vi "Write Loop.vi"(7 "Enum - Menu":enum16{"INIT", "WRITE", "RE-INIT", "CLOSE"}(ring), 8 "error in (no error)":errorcluster, 11 "Uplink Packet":T1) -> (0 "error out":errorcluster)   [LabVIEW 2025]
panel:
  out "connection ID":refnum<k16>
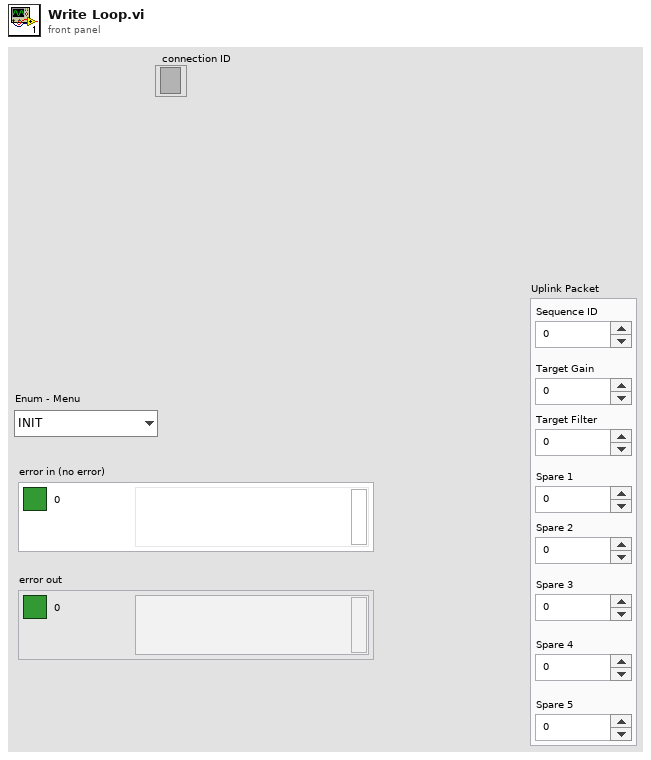
[diagram p1: front panel]
types:
  T1 = cluster{"Sequence ID":u32, "Target Gain":u32, "Target Filter":u32, "Spare 1":u32, "Spare 2":u32, "Spare 3":u32, "Spare 4":u32, "Spare 5":u32}
  T2 = enum16{"big-endian, network order", "native, host order", "little-endian"}
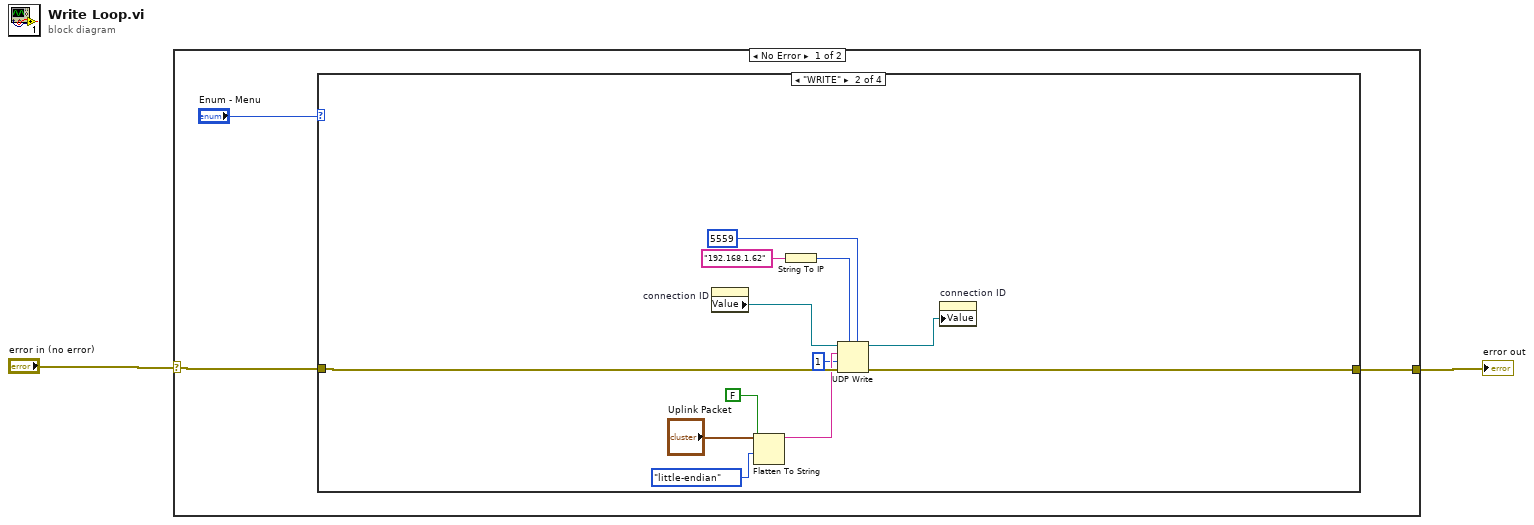
[diagram p0: block diagram]
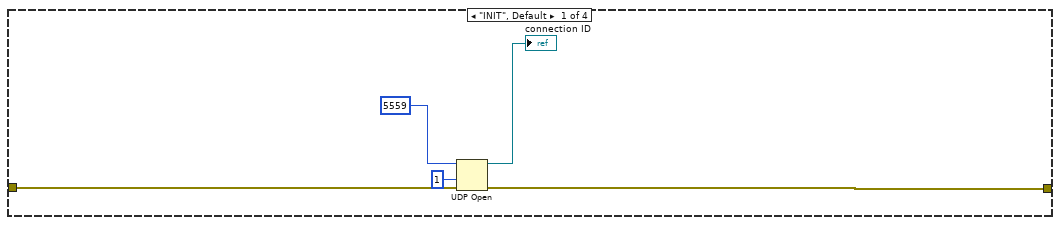
[diagram p2: hidden frame]
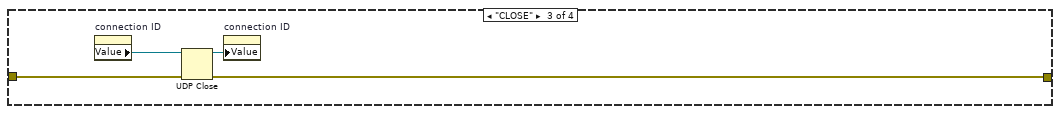
[diagram p3: hidden frame]
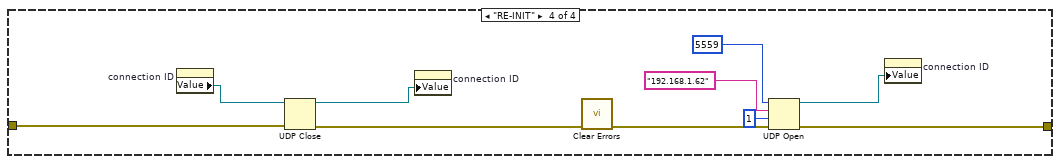
[diagram p4: hidden frame]
diagram:
  n1 = case shown="No Error" "error in (no error)" {
    selector: "error in (no error)" -> [w4 _]
    tunnel: [w3 _] -> w1
    frame No Error {
      n2 = case shown="\"WRITE\"" "Enum - Menu" {
        tunnel: w4 -> [w9 w21 w24 w36]
        tunnel: [w8 w20 w23 w30] -> w3
        frame "INIT", Default {
          n3 = UDP Open(8:w9, 9:1 ("timeout ms (25000)"), 11:u16 5559 ("port")) -> (port=→"connection ID":refnum<k16>, 0:w8:errorcluster)  [unwired: 2 in, 1 out]
        }
        frame "WRITE" {
          n4 = property on="connection ID" class="Ref (strict)"() -> ("Value"=w17:refnum<k16>)  [unwired: 2 in, 2 out]
          n5 = Flatten To String(anything="Uplink Packet", prepend array or string size? (T)=FALSE, byte order (0:big-endian, network order)=T2."little-endian") -> (data string=w12:string)  [unwired: 1 in, 2 out]
          n6 = String To IP(1:"192.168.1.62" ("name")) -> (0:w22:u32)
          n7 = UDP Write(address=w22, port or service name=u16 5559, connection ID=w17, data in=w12, 8:w21, 9:1 ("timeout ms (25000)")) -> (error out=w20:errorcluster, 3:w16:refnum<k16>)
          n8 = property on="connection ID" class="Ref (strict)"("Value"=w16) -> ()  [unwired: 2 in, 2 out]
        }
        frame "CLOSE" {
          n9 = property on="connection ID" class="Ref (strict)"() -> ("Value"=w26:refnum<k16>)  [unwired: 2 in, 2 out]
          n10 = UDP Close(connection ID=w26, 8:w24) -> (connection ID out=w25:refnum<k16>, error out=w23:errorcluster)
          n11 = property on="connection ID" class="Ref (strict)"("Value"=w25) -> ()  [unwired: 2 in, 2 out]
        }
        frame "RE-INIT" {
          n12 = property on="connection ID" class="Ref (strict)"() -> ("Value"=w35:refnum<k16>)  [unwired: 2 in, 2 out]
          n13 = UDP Close(connection ID=w35, 8:w36) -> (connection ID out=w34:refnum<k16>, error out=w31:errorcluster)
          n14 = property on="connection ID" class="Ref (strict)"("Value"=w34) -> ()  [unwired: 2 in, 2 out]
          n15 = call <vilib>:"Clear Errors.vi"("error in (no error)"=w31) -> ("error out"=w28:errorcluster)  [unwired: 5 in, 1 out]
          n16 = UDP Open(8:w28, 9:1 ("timeout ms (25000)"), 10:"192.168.1.62" ("service name"), 11:u16 5559 ("port")) -> (port=w29:refnum<k16>, 0:w30:errorcluster)  [unwired: 1 in, 1 out]
          n17 = property on="connection ID" class="Ref (strict)"("Value"=w29) -> ()  [unwired: 2 in, 2 out]
        }
      }
    }
    frame Error {
    }
  }
  "error out" <- w1
